vi "ExXCamGSameGraph.vi"() -> ()   [LabVIEW 2010]
uses:
  GlbCamHndls.vi
panel:
  in  "Number of Cameras":u32=1 min=1 max=20 step=1
  out "Camera 16":sgl[](graph)
  out "Camera 15":sgl[](graph)
  out "Camera 14":sgl[](graph)
  out "Camera 13":sgl[](graph)
  out "Camera 12":sgl[](graph)
  out "Camera 11":sgl[](graph)
  out "Camera 10":sgl[](graph)
  out "Camera 9":sgl[](graph)
  out "Camera 8":sgl[](graph)
  out "Camera 7":sgl[](graph)
  out "Camera 6":sgl[](graph)
  out "Camera 5":sgl[](graph)
  out "Camera 4":sgl[](graph)
  out "Camera 3":sgl[](graph)
  out "Camera 2":sgl[](graph)
  out "Camera 1":sgl[](graph)
  in  "stop":bool
  in  "Exposure":dbl=0.5 format="%.2f"
  out "error out":errorcluster
  in  "error in (no error)":errorcluster
  # "Ex2CamerasSameGraph:\nThis example runs two cameras in focus mode.\nSets them up for center strip and displays as graph.\nRemember to setup two cameras in the pvcam.ini\nfile."
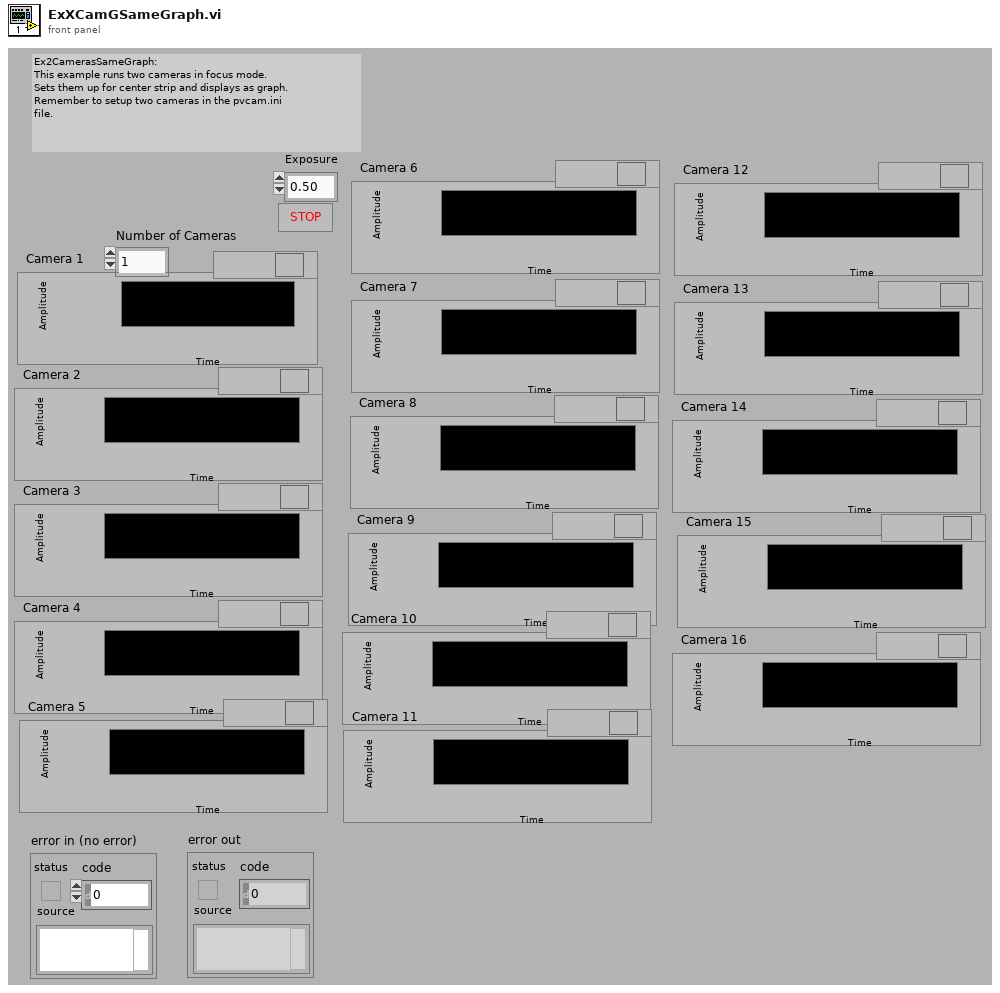
[diagram p1: front panel]
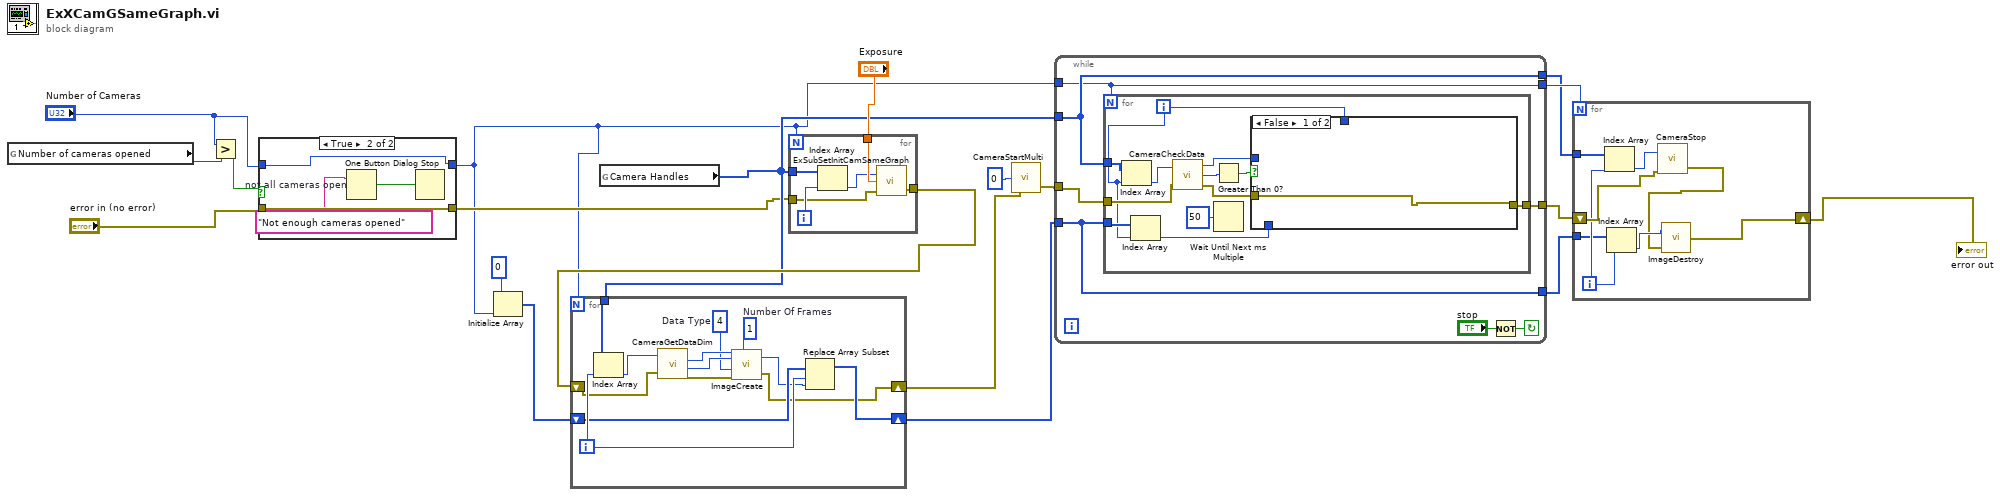
[diagram p0: block diagram]
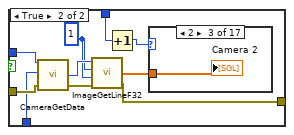
[diagram p3: hidden frame]
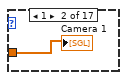
[diagram p5: hidden frame]
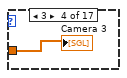
[diagram p6: hidden frame]
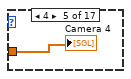
[diagram p7: hidden frame]
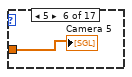
[diagram p8: hidden frame]
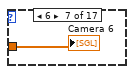
[diagram p9: hidden frame]
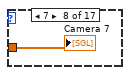
[diagram p10: hidden frame]
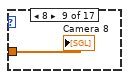
[diagram p11: hidden frame]
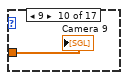
[diagram p12: hidden frame]
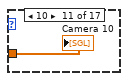
[diagram p13: hidden frame]
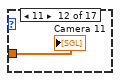
[diagram p14: hidden frame]
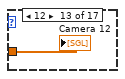
[diagram p15: hidden frame]
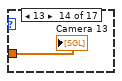
[diagram p16: hidden frame]
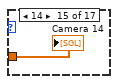
[diagram p17: hidden frame]
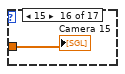
[diagram p18: hidden frame]
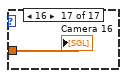
[diagram p19: hidden frame]
diagram:
  n1 = global read "GlbCamHndls.vi" "Number of cameras opened"() -> (w2:u32)
  n2 = Greater?(x="Number of Cameras", y=w2) -> (0:w6:bool)
  n3 = case shown="True" w6 {
    tunnel: "error in (no error)" -> [w22 w26]
    tunnel: [w22 w26] -> w4
    tunnel: "Number of Cameras" -> [w21 w25]
    tunnel: [w21 w25] -> w3
    frame False {
    }
    frame True {
      n4 = One Button Dialog "not all cameras open"(message="Not enough cameras opened") -> (true=w24:bool)  [unwired: 1 in]
      n5 = Stop(stop? (T)=w24) -> ()
    }
  }
  n6 = Initialize Array(0, w3) -> (w16:i32[])
  n7 = global read "GlbCamHndls.vi" "Camera Handles"() -> (w8:u32[])
  n8 = for {
    N: w3 -> [_]
    tunnel: w8 -> [w32]
    tunnel: w4 -> [w28]
    tunnel: [w30] -> w15
    tunnel: "Exposure" -> [w29]
    i -> [w31]
    n9 = Index Array(array=w32, index=w31) -> (element=w27:u32)
    n10 = call "ExSubSetInitCamSameGraph.vi"("error in (no error)"=w28, "Exposure"=w29, "Camera Handle"=w27) -> ("error out"=w30:errorcluster)  [unwired: 1 out]
  }
  n11 = for {
    N: w3 -> [_]
    shift-right: [w34] -> w13
    shift-left: w16 -> [w36]
    shift-right: [w33] -> w14
    shift-left: w15 -> [w42]
    tunnel: w8 -> [w45]
    i -> [w44]
    w40 = u32 1  # Number Of Frames
    w37 = u32 4  # Data Type
    n12 = Index Array(array=w45, index=w44) -> (element=w43:u32)
    n13 = call <userlib>:"CameraGetDataDim.vi"("Camera Handle"=w43, "error in"=w42) -> ("Xdim"=w39:u32, "Ydim"=w38:u32, "error out"=w41:errorcluster)  [unwired: 1 out]
    n14 = call <userlib>:"ImageCreate.vi"("X dimension"=w39, "Y dimension"=w38, "Data Type"=w37, "error in"=w41, "Number Of Frames"=w40) -> ("Image Handle"=w35:u32, "error out"=w33:errorcluster)
    n15 = Replace Array Subset(array=w36, new element=w35, index=w44) -> (w34:i32[])
  }
  n16 = call "CameraStartMulti.vi"("error in (no error)"=w14, "Number Of Cameras"=0) -> ("error out"=w19:errorcluster)  [unwired: 1 in, 1 out]
  n17 = while {
    tunnel: w19 -> [w50]
    tunnel: w8 -> [w48]
    tunnel: [w49] -> w9
    tunnel: w3 -> [w46]
    tunnel: w13 -> [w47]
    tunnel: [w48] -> w11
    tunnel: [w47] -> w10
    tunnel: [w46] -> w12
    stop <- w51 continue-if-true
    n18 = for {
      N: w46 -> [_]
      tunnel: [w59] -> w49
      tunnel: w48 -> [w58]
      tunnel: w50 -> [w56]
      tunnel: w47 -> [w55]
      i -> [w53]
      n19 = Index Array(array=w58, index=w53) -> (element=w57:u32)
      n20 = Index Array(array=w55, index=w53) -> (element=w54:i32)
      n21 = call <userlib>:"CameraCheckData.vi"("Camera Handle"=w57, "error in"=w56) -> ("Camera Handle"=w61:u32, "Number Of Frames Available"=w63:i32, "error out"=w60:errorcluster)
      n22 = Greater Than 0?(x=w63) -> (x > 0?=w62:bool)
      n23 = Wait Until Next ms Multiple(millisecond multiple=u32 50) -> ()  [unwired: 1 out]
      n24 = case shown="False" w62 {
        tunnel: [w65 w72] -> w59
        tunnel: w61 -> [_ w71]
        tunnel: w60 -> [w65 w70]
        tunnel: w53 -> [_ w66]
        tunnel: w54 -> [_ w68]
        frame False {
        }
        frame True {
          w73 = 1
          n25 = call <userlib>:"CameraGetData.vi"("error in"=w70, "Data Handle"=w68, "Camera Handle"=w71) -> ("error out"=w75:errorcluster, "Data Handle"=w74:u32)  [unwired: 1 out]
          n26 = call <userlib>:"ImageGetLineF32.vi"("error in"=w75, "Z Position"=w73, "Y Position"=w73, "Data Handle"=w74) -> ("error out"=w72:errorcluster, "Array F32"=w69:sgl[])  [unwired: 1 out]
          n27 = Increment(x=w66) -> (x+1=w67:i32)
          n28 = case shown="2" w67 {
            tunnel: w69 -> [_ w76 w77 w78 w79 w80 w81 w82 w83 w84 w85 w86 w87 w88 w89 w90 w91]
            frame Default {
            }
            frame 1 {
              "Camera 1" <- w76
            }
            frame 2 {
              "Camera 2" <- w77
            }
            frame 3 {
              "Camera 3" <- w78
            }
            frame 4 {
              "Camera 4" <- w79
            }
            frame 5 {
              "Camera 5" <- w80
            }
            frame 6 {
              "Camera 6" <- w81
            }
            frame 7 {
              "Camera 7" <- w82
            }
            frame 8 {
              "Camera 8" <- w83
            }
            frame 9 {
              "Camera 9" <- w84
            }
            frame 10 {
              "Camera 10" <- w85
            }
            frame 11 {
              "Camera 11" <- w86
            }
            frame 12 {
              "Camera 12" <- w87
            }
            frame 13 {
              "Camera 13" <- w88
            }
            frame 14 {
              "Camera 14" <- w89
            }
            frame 15 {
              "Camera 15" <- w90
            }
            frame 16 {
              "Camera 16" <- w91
            }
          }
        }
      }
    }
    n29 = Not(x="stop") -> (.not. x?=w51:bool)
  }
  n30 = for {
    N: w12 -> [_]
    shift-right: [w99] -> w7
    shift-left: w9 -> [w98]
    tunnel: w11 -> [w96]
    tunnel: w10 -> [w95]
    i -> [w97]
    n31 = Index Array(array=w96, index=w97) -> (element=w93:u32)
    n32 = Index Array(array=w95, index=w97) -> (element=w94:i32)
    n33 = call <userlib>:"CameraStop.vi"("error in"=w98, "Camera Handle"=w93) -> ("error out"=w92:errorcluster)  [unwired: 1 out]
    n34 = call <userlib>:"ImageDestroy.vi"("error in"=w92, "Data handle"=w94) -> ("error out"=w99:errorcluster)
  }
  "error out" <- w7
